vi "Get Arguments as LabVIEW Data.vi"(7 "type":variant, 8 "error in (no error)":errorcluster, 11 "Call in":refnum<class "Call.lvclass">) -> (0 "error out":errorcluster, 2 "LabVIEW Data":variant, 3 "Call out":refnum<class "Call.lvclass">)   [LabVIEW 2013, in "JKI_Python_Bridge_for_LV.lvlib" / "Call.lvclass"]
uses:
  Call.lvclass
  Call.lvclass/Call.ctl
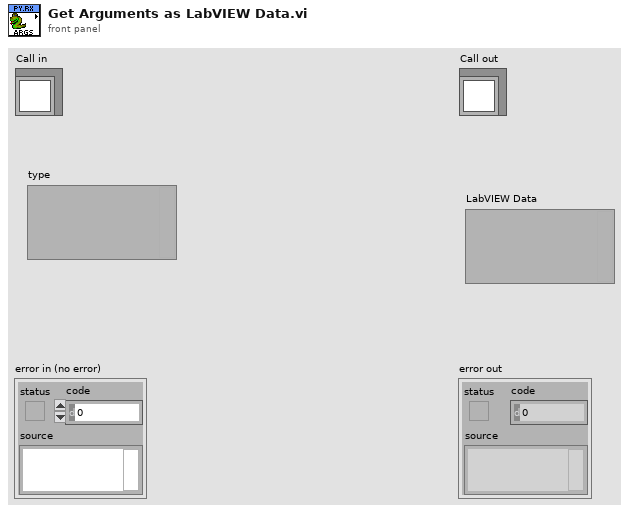
[diagram p1: front panel]
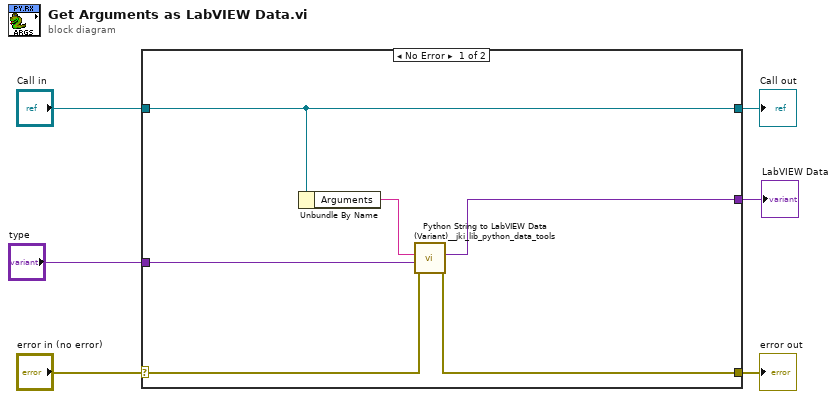
[diagram p0: block diagram]
diagram:
  n1 = case shown="No Error" "error in (no error)" {
    selector: "error in (no error)" -> [w10 w14]
    tunnel: [w9 w14] -> w5
    tunnel: [w12 w13] -> w3
    tunnel: "Call in" -> [w12 w13]
    tunnel: [w7 _] -> w2
    tunnel: "type" -> [w11 _]
    frame No Error {
      n2 = Unbundle By Name(w12) -> ("Arguments"=w8:string)
      n3 = call <vilib>:"Python String to LabVIEW Data (Variant)__jki_lib_python_data_tools.vi"("error in (no error)"=w10, "type"=w11, "Python String"=w8) -> ("error out"=w9:errorcluster, "LabVIEW Data"=w7:variant)  [unwired: 7 in]
    }
    frame Error {
    }
  }
  "error out" <- w5
  "Call out" <- w3
  "LabVIEW Data" <- w2
